vi "Update Tree Items.vi"(8 "error in (no error)":errorcluster, 10 "Tree Control Item":T1(array[cluster]), 11 "ICD System Tree View in":refnum<class "[V]System Tree View.lvclass">) -> (0 "error out":errorcluster, 3 "ICD System Tree View out":refnum<class "[V]System Tree View.lvclass">)   [LabVIEW 2020, in "[V]System Tree View.lvlib" / "[V]System Tree View.lvclass"]
uses:
  [V]System Tree View.lvclass
  [V]System Tree View.lvclass/[V]System Tree View.ctl
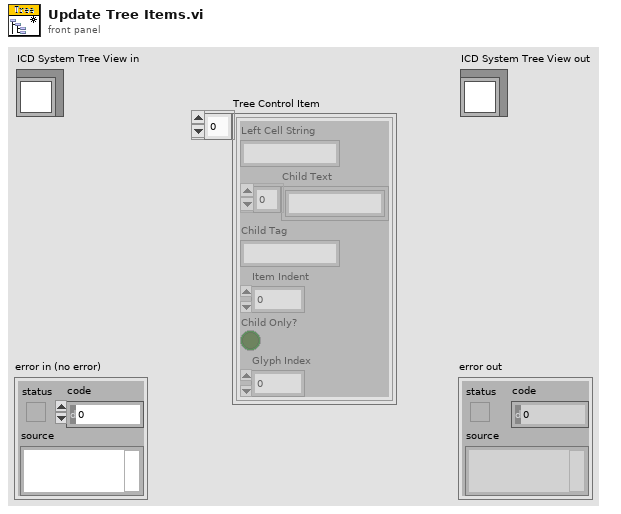
[diagram p1: front panel]
types:
  T1 = cluster{"Left Cell String":string, "Child Text":string[], "Child Tag":string, "Item Indent":i32, "Child Only?":bool, "Glyph Index":i32}[]
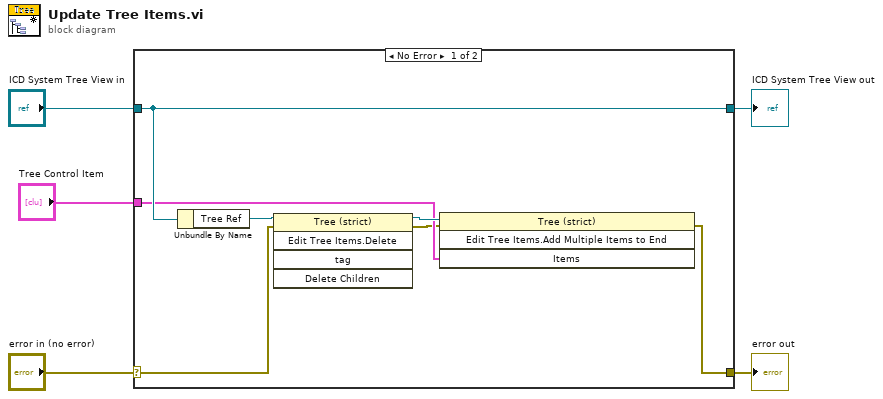
[diagram p0: block diagram]
diagram:
  n1 = case shown="No Error" "error in (no error)" {
    selector: "error in (no error)" -> [w8 w14]
    tunnel: [w6 w14] -> w4
    tunnel: [w12 w13] -> w2
    tunnel: "ICD System Tree View in" -> [w12 w13]
    tunnel: "Tree Control Item" -> [w9 _]
    frame No Error {
      n2 = Unbundle By Name(w12) -> ("Tree Ref"=w11:refnum<vi>)
      n3 = invoke class="Tree (strict)" method="Edit Tree Items.Delete"(reference=w11, error in=w8) -> (reference out=w10:refnum<vi>, error out=w7:errorcluster)  [unwired: 3 in, 3 out]
      n4 = invoke class="Tree (strict)" method="Edit Tree Items.Add Multiple Items to End"(reference=w10, error in=w7, "Items"=w9) -> (error out=w6:errorcluster)  [unwired: 1 in, 3 out]
    }
    frame Error {
    }
  }
  "error out" <- w4
  "ICD System Tree View out" <- w2
